vi "Determine Warnings VI Exercise 3-9.vi"() -> ()   [LabVIEW 2014]
panel:
  in  "Max Wind Speed":dbl
  in  "Current Wind Speed":dbl
  out "Warning?":bool
  out "Warning Text":string
  in  "Min Temp":dbl
  in  "Max Temp":dbl
  in  "Current Temp":dbl
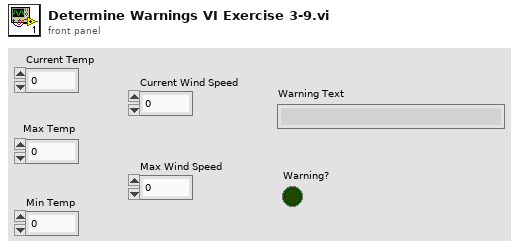
[diagram p1: front panel]
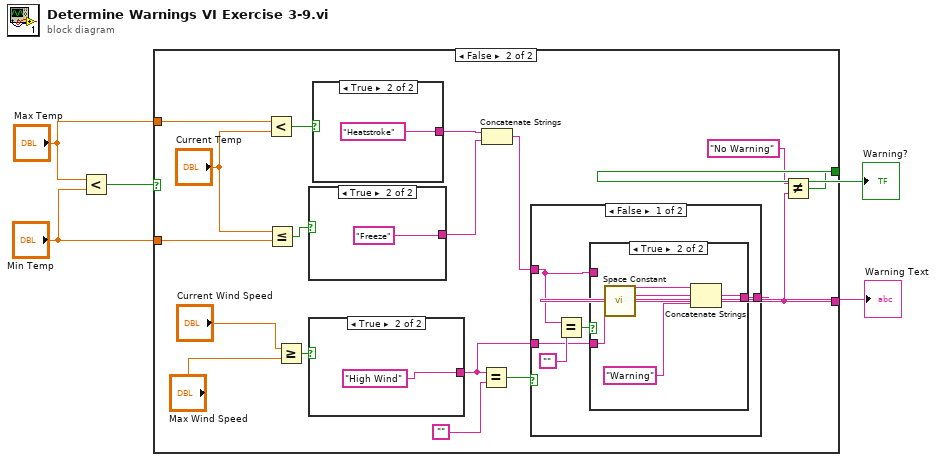
[diagram p0: block diagram]
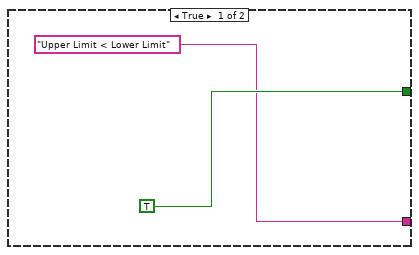
[diagram p2: hidden frame]
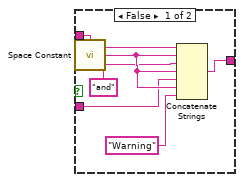
[diagram p3: hidden frame]
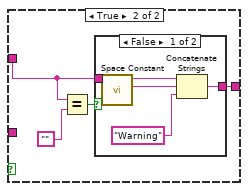
[diagram p4: hidden frame]
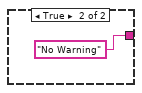
[diagram p5: hidden frame]
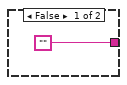
[diagram p7: hidden frame]
diagram:
  n1 = Less?(x="Max Temp", y="Min Temp") -> (x < y?=w4:bool)
  n2 = case shown="False" w4 {
    tunnel: [TRUE w11] -> w5
    tunnel: ["Upper Limit < Lower Limit" w9] -> w1
    tunnel: "Max Temp" -> [_ w24]
    tunnel: "Min Temp" -> [_ w22]
    frame True {
    }
    frame False {
      n3 = Less?(x=w24, y="Current Temp") -> (x < y?=w21:bool)
      n4 = Less Or Equal?(x="Current Temp", y=w22) -> (x <= y?=w18:bool)
      n5 = Greater Or Equal?(x="Current Wind Speed", y="Max Wind Speed") -> (x >= y?=w17:bool)
      n6 = case shown="True" w18 {
        tunnel: ["" "Freeze"] -> w19
        frame False {
        }
        frame True {
        }
      }
      n7 = case shown="True" w17 {
        tunnel: [_ "High Wind"] -> w13
        frame False {
        }
        frame True {
        }
      }
      n8 = case shown="True" w21 {
        tunnel: [_ "Heatstroke"] -> w20
        frame False {
        }
        frame True {
        }
      }
      n9 = Equal?(x=w13, y="") -> (x = y?=w14:bool)
      n10 = Concatenate Strings(w20, w19) -> (w12:string)
      n11 = case shown="False" w14 {
        tunnel: w13 -> [w26 _]
        tunnel: w12 -> [w27 w42]
        tunnel: [w25 w41] -> w9
        frame False {
          n12 = Equal?(x=w27, y="") -> (x = y?=w29:bool)
          n13 = case shown="True" w29 {
            tunnel: w27 -> [w35 _]
            tunnel: w26 -> [w32 w38]
            tunnel: [w30 w39] -> w25
            frame False {
              n14 = call <vilib>:"Space Constant.vi"() -> ("String"=w34:string)
              n15 = Concatenate Strings(w35, w34, "and", w34, w32, w34, "Warning") -> (w30:string)
            }
            frame True {
              n16 = call <vilib>:"Space Constant.vi"() -> ("String"=w37:string)
              n17 = Concatenate Strings(w38, w37, "Warning") -> (w39:string)
            }
          }
        }
        frame True {
          n18 = Equal?(x=w42, y="") -> (x = y?=w43:bool)
          n19 = case shown="False" w43 {
            tunnel: w42 -> [w47 _]
            tunnel: [w44 "No Warning"] -> w41
            frame False {
              n20 = call <vilib>:"Space Constant.vi"() -> ("String"=w45:string)
              n21 = Concatenate Strings(w47, w45, "Warning") -> (w44:string)
            }
            frame True {
            }
          }
        }
      }
      n22 = Not Equal?(x="No Warning", y=w9) -> (x != y?=w11:bool)
    }
  }
  "Warning Text" <- w1
  "Warning?" <- w5
